vi "EndTestSuite_AfterSiblingFailure_PassedIconSet.vi"() -> (0 "error out":errorcluster)   [LabVIEW 2017, in "ResultTreeListener.Tests.lvlib"]
uses:
  ResultTreeListener.Tests.lvlib
  ResultTree/Icon.ctl
  275d98eb-69a7-4435-8809-2af3ffd1cf1d.vi
  Support/FakeTestSuite/FakeTestSuite.lvclass
  C:/Users/de200256/Code/logmanoriginal/lvunit/TestSuite/TestSuite.lvclass
  Support/FakeTestCase/FakeTestCase.lvclass
  C:/Users/de200256/Code/logmanoriginal/lvunit/Test/Test.lvclass
  Constraint/IsEqual/Create.vi
  ResultTreeListener/ResultTreeListener.lvclass
  Constraint/IsEqual/IsEqual.lvclass
  ResultTree/ResultTree.lvclass
panel:
  in  "Tree":string(tree)
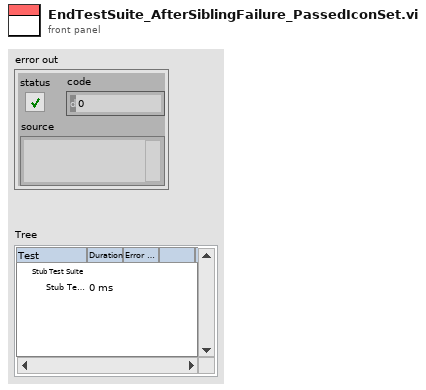
[diagram p1: front panel]
types:
  T1 = typedef "ResultTree.lvclass/Icon.ctl" = enum16{"None", "Passed", "Failed", "Error"}
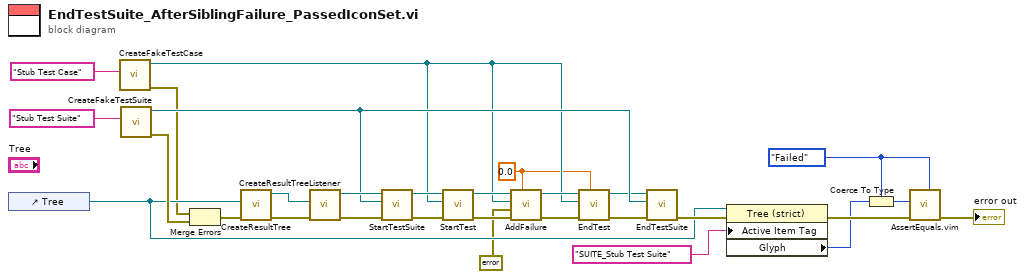
[diagram p0: block diagram]
diagram:
  w1 = 0.0 ("Time")
  w14 = Icon."Failed" ("Active Cell:String")
  n1 = control-ref of="Tree"() -> (w18:refnum<vi>)
  n2 = call "CreateFakeTestCase.vi"("Name"="Stub Test Case") -> ("error out"=w12:errorcluster, "FakeTestCase out"=w2:refnum<class "FakeTestCase.lvclass">)  [unwired: 9 in]
  n3 = call "CreateFakeTestSuite.vi"("Name"="Stub Test Suite") -> ("error out"=w22:errorcluster, "FakeTestSuite out"=w20:refnum<class "FakeTestSuite.lvclass">)  [unwired: 9 in]
  n4 = Merge Errors(w12, w22) -> (w13:errorcluster)
  n5 = call "CreateResultTree.vi"("error in (no error)"=w13, "Tree Refnum"=w18) -> ("error out"=w29:errorcluster, "ResultTree out"=w28:refnum<class "ResultTree.lvclass">)  [unwired: 8 in]
  n6 = call "CreateResultTreeListener.vi"("error in (no error)"=w29, "ResultTree"=w28) -> ("error out"=w27:errorcluster, "ResultTreeListener out"=w25:refnum<class "ResultTreeListener.lvclass">)  [unwired: 8 in]
  n7 = call-dynamic "StartTestSuite.vi"("error in (no error)"=w27, "TestSuite"=w20, "ResultTreeListener in"=w25) -> ("error out"=w23:errorcluster, "ResultTreeListener out"=w10:refnum<class "ResultTreeListener.lvclass">)  [unwired: 7 in]
  n8 = call-dynamic "StartTest.vi"("error in (no error)"=w23, "Test"=w2, "ResultTreeListener in"=w10) -> ("error out"=w8:errorcluster, "ResultTreeListener out"=w7:refnum<class "ResultTreeListener.lvclass">)  [unwired: 7 in]
  n9 = call-dynamic "AddFailure.vi"("Time"=w1, "error in (no error)"=w8, "Failure"=errorcluster {"status"=TRUE, "code"=1, "source"="Error."}, "Test"=w2, "ResultTreeListener in"=w7) -> ("error out"=w9:errorcluster, "ResultTreeListener out"=w4:refnum<class "ResultTreeListener.lvclass">)  [unwired: 5 in]
  n10 = call-dynamic "EndTest.vi"("Time"=w1, "error in (no error)"=w9, "Test"=w2, "ResultTreeListener in"=w4) -> ("error out"=w5:errorcluster, "ResultTreeListener out"=w3:refnum<class "ResultTreeListener.lvclass">)  [unwired: 6 in]
  n11 = call-dynamic "EndTestSuite.vi"("error in (no error)"=w5, "TestSuite"=w20, "ResultTreeListener in"=w3) -> ("error out"=w21:errorcluster)  [unwired: 7 in, 1 out]
  n12 = property class="Tree (strict)"(reference=w18, error in=w21, "Active Item Tag"="SUITE_Stub Test Suite" ("Active Item:Tag")) -> (error out=w19:errorcluster, "Glyph"=w16:i32)  [unwired: 1 out]
  n13 = Coerce To Type(0:w16, 1:w14) -> (2:w15:T1)
  n14 = call "AssertEquals.vim"("Expected"=w14, "error in (no error)"=w19, "Actual"=w15) -> ("error out"=→"error out":errorcluster)  [unwired: 8 in]
